vi "UI Set Tree Selection.vi"(8 "error in (no error)":errorcluster, 10 "Tag in (TopLeft)":string, 11 "Controller in":refnum<class "Controller.lvclass">) -> (0 "error out":errorcluster, 2 "Tag out":string, 3 "Controller out":refnum<class "Controller.lvclass">)   [LabVIEW 2013, in "SET Project Editor.lvlib" / "Controller.lvclass"]
uses:
  Controller.lvclass
  Controller.lvclass/Controller.ctl
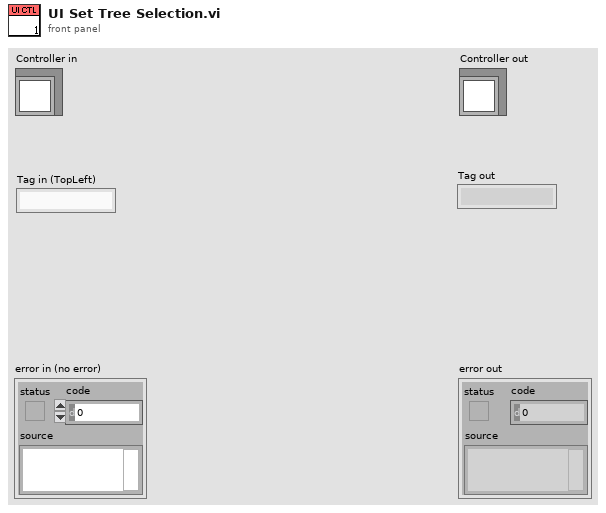
[diagram p1: front panel]
types:
  T1 = typedef "LVNodeAndColumnTypeDef.ctl" = cluster{"Node":string, "Column":i32}
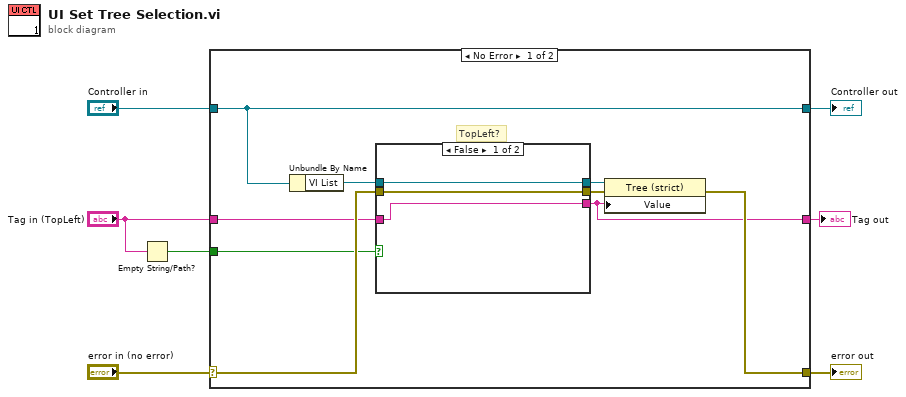
[diagram p0: block diagram]
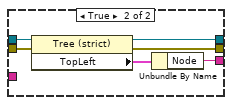
[diagram p2: hidden frame]
diagram:
  n1 = Empty String/Path?(string/path="Tag in (TopLeft)") -> (empty?=w2:bool)
  n2 = case shown="No Error" "error in (no error)" {
    selector: "error in (no error)" -> [w13 w28]
    tunnel: [w11 w28] -> w6
    tunnel: [w16 w27] -> w4
    tunnel: "Controller in" -> [w16 w27]
    tunnel: "Tag in (TopLeft)" -> [w9 w26]
    tunnel: w2 -> [w10 _]
    tunnel: [w8 w26] -> w1
    frame No Error {
      # "TopLeft?"
      n3 = Unbundle By Name(w16) -> ("VI List"=w15:refnum<vi>)
      n4 = case shown="False" w10 {
        tunnel: w15 -> [w18 w25]
        tunnel: [w18 w23] -> w14
        tunnel: [w19 w22] -> w8
        tunnel: w13 -> [w17 w21]
        tunnel: [w17 w20] -> w12
        tunnel: w9 -> [w19 _]
        frame False {
        }
        frame True {
          n5 = property class="Tree (strict)"(reference=w25, error in=w21) -> (reference out=w23:refnum<vi>, error out=w20:errorcluster, "TopLeft"=w24:T1)
          n6 = Unbundle By Name(w24) -> ("Node"=w22:string)
        }
      }
      n7 = property class="Tree (strict)"(reference=w14, error in=w12, "Value"=w8) -> (error out=w11:errorcluster)  [unwired: 1 out]
    }
    frame Error {
    }
  }
  "error out" <- w6
  "Controller out" <- w4
  "Tag out" <- w1
